vi "Launch HAL Actor.vi"(8 "error in (no error)":errorcluster, 11 "App Actor in":refnum<class "App Actor.lvclass">) -> (0 "error out":errorcluster, 3 "App Actor out":refnum<class "App Actor.lvclass">)   [LabVIEW 2024, in "App Actor.lvlib" / "App Actor.lvclass"]
uses:
  App Actor.lvclass
  App Actor.lvclass/App Actor.ctl
  <vilib>/ActorFramework/Actor/Actor.lvclass
  HAL Interface Actor/HAL Interface Actor/HAL Interface Actor.lvclass
  C:/Program Files (x86)/National Instruments/LabVIEW 2024/vi.lib/ActorFramework/Actor/Actor.lvclass
  C:/Users/cuswsf/Desktop/App Actor/HAL Interface Actor/HAL Interface Actor/HAL Interface Actor.lvclass
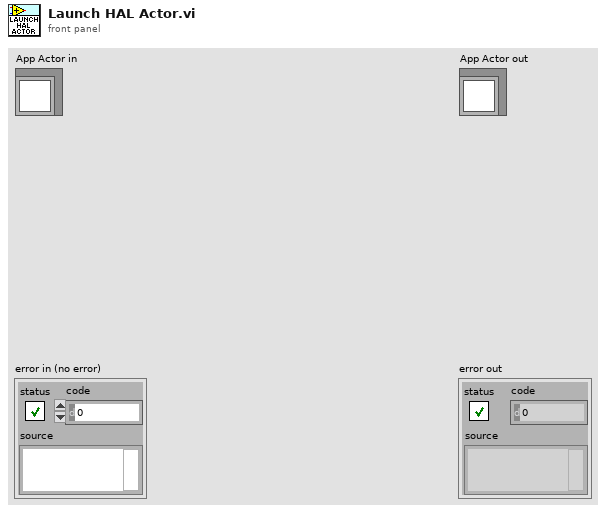
[diagram p1: front panel]
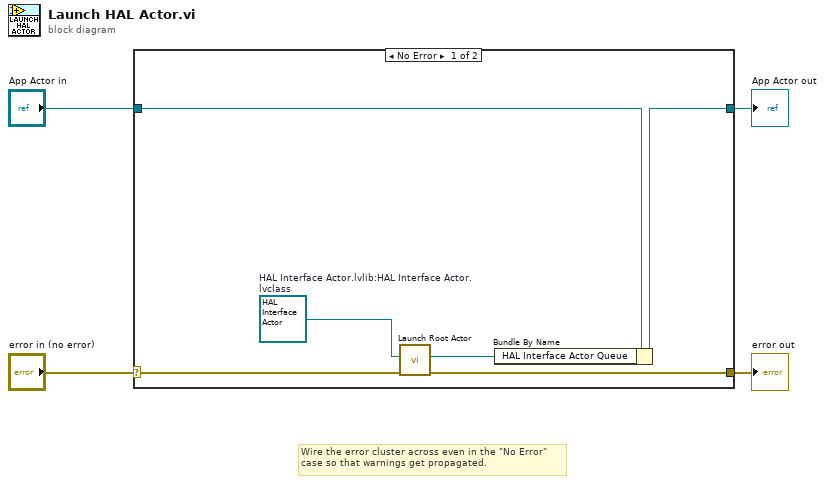
[diagram p0: block diagram]
diagram:
  # "Wire the error cluster across even in the \"No Error\"\ncase so that warnings get propagated."
  n1 = case shown="No Error" "error in (no error)" {
    selector: "error in (no error)" -> [w9 w12]
    tunnel: [w8 w12] -> w3
    tunnel: [w6 w11] -> w1
    tunnel: "App Actor in" -> [w10 w11]
    frame No Error {
      w7 = refnum<class "HAL Interface Actor.lvclass"> refnum  # HAL Interface Actor.lvlib:HAL Interface Actor.lvclass
      n2 = call <vilib>:"Launch Root Actor.vi"("error in (no error)"=w9, "Actor"=w7) -> ("error out"=w8:errorcluster, "Actor's Enqueuer"=w5:refnum<class "Message Enqueuer.lvclass">)  [unwired: 8 in]
      n3 = Bundle By Name(cluster=w10, "HAL Interface Actor Queue"=w5) -> (w6:refnum<class "App Actor.lvclass">)
    }
    frame Error {
    }
  }
  "error out" <- w3
  "App Actor out" <- w1
